vi "EnFloHubRunning.vi"() -> (2 "EnFloHubRunning":bool)   [LabVIEW 2020]
uses:
  Anemometry Sub Vis/Globals/Dynamic_call_global.ph.vi
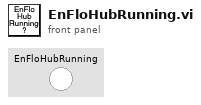
[diagram p1: front panel]
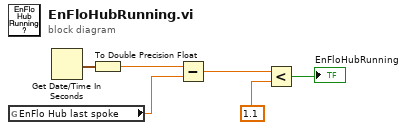
[diagram p0: block diagram]
diagram:
  n1 = global read "Dynamic_call_global.ph.vi" "EnFlo Hub last spoke"() -> (w5:dbl)
  n2 = Get Date/Time In Seconds() -> (seconds since 1Jan1904=w6:timestamp)
  n3 = To Double Precision Float(number=w6) -> (double precision float=w4:dbl)
  n4 = Subtract(x=w4, y=w5) -> (x-y=w3:dbl)
  n5 = Less?(x=w3, y=1.1) -> (x < y?=→"EnFloHubRunning":bool)
